vi "Initialize Scope and FGEN with Tclk.vi"(7 "Tclk Boolean Ref":refnum<vi>, 10 "FGEN Resources in":refnum<k15>[](array[refnum])=["FGEN1", "FGEN2"], 11 "Scope Resources in":refnum<k15>[](array[refnum])=["SCOPE1", "SCOPE2"]) -> (0 "error out":errorcluster, 1 "Tclk Refs Array":refnum<k20>[](array[refnum]), 2 "FGEN Resources out":refnum<k15>[](array[refnum]), 3 "Scope Resources out":refnum<k15>[](array[refnum]), 5 "scope channels":string[](array[string]))   [LabVIEW 2024]
uses:
  <instrlib>/niFgen/niFgen.llb/niFgen Output Mode.ctl
  <instrlib>/niFgen/niFgen.llb/niFgen Trigger Mode.ctl
  <instrlib>/niScope/Controls/niScope trigger source.ctl
  <instrlib>/niFgen/niFgen.llb/niFgen Create Waveform (WDT).vi
  <instrlib>/niScope/Configure/Trigger/niScope Configure Trigger Edge.vi
panel:
  out "Preparing T-Clk":bool
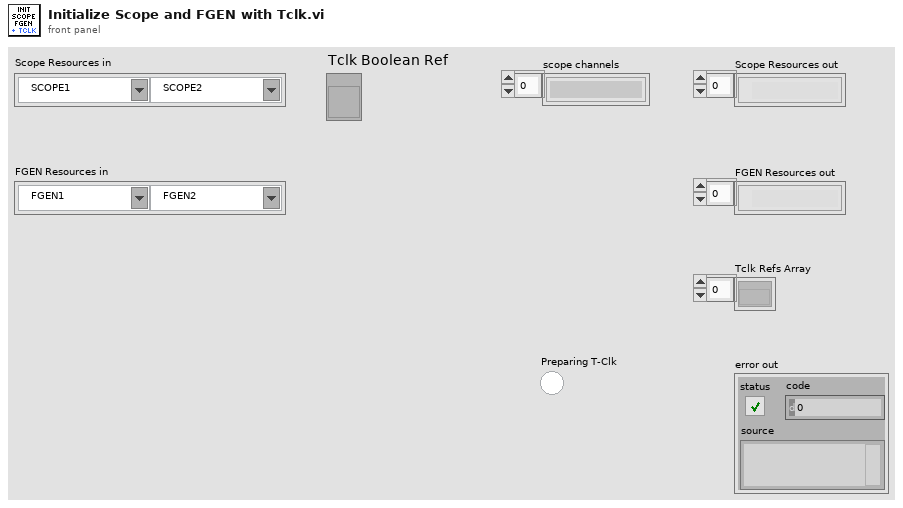
[diagram p1: front panel]
types:
  T1 = typedef "niScope trigger source.ctl" = string
  T2 = typedef "niFgen Trigger Mode.ctl" = i32
  T3 = typedef "niFgen Output Mode.ctl" = u32
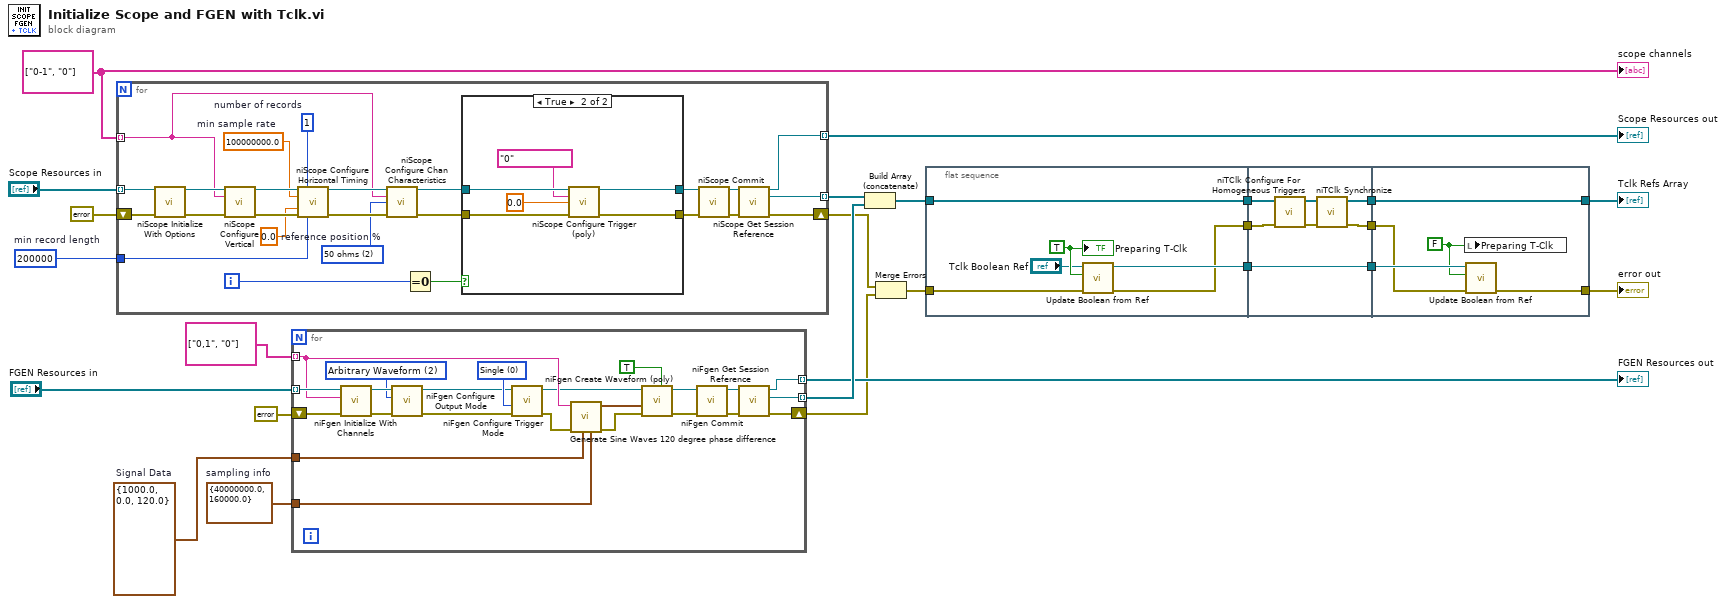
[diagram p0: block diagram]
diagram:
  w17 = 200000  # min record length
  w16 = cluster{"f":dbl, "startPhase":dbl, "dPhase":dbl} {"f"=1000.0, "startPhase"=0.0, "dPhase"=120.0}  # Signal Data
  w18 = cluster{"Fs":dbl, "#s":dbl} {"Fs"=40000000.0, "#s"=160000.0}  # sampling info
  w9 = string[] ["0-1", "0"] ("channels")
  n1 = for {
    tunnel: [w44] -> w15 mode=indexing
    tunnel: "Scope Resources in" -> [w35] mode=indexing
    tunnel: [w41] -> w6 mode=indexing
    tunnel: w9 -> [w27] mode=indexing
    shift-right: [w40] -> w1
    shift-left: errorcluster {"status"=FALSE, "code"=0, "source"=""} ("error out") -> [w39]
    tunnel: w17 -> [w26]
    i -> [w42]
    w28 = u32 2 items=["1 mega ohm"=0, "50 ohms"=2] ("input impedance")
    w36 = 0.0  # reference position %
    w37 = 1  # number of records
    w38 = 100000000.0  # min sample rate
    n2 = call <instrlib>:"niScope Initialize With Options.vi"("resource name"=w35, "error in"=w39) -> ("instrument handle"=w48:refnum<k15>, "error out"=w47:errorcluster)  [unwired: 12 in]
    n3 = call <instrlib>:"niScope Configure Vertical.vi"("instrument handle"=w48, "channels"=w27, "error in"=w47) -> ("instrument handle out"=w46:refnum<k15>, "error out"=w45:errorcluster)  [unwired: 11 in]
    n4 = call <instrlib>:"niScope Configure Horizontal Timing.vi"("instrument handle"=w46, "number of records"=w37, "min sample rate"=w38, "reference position"=w36, "error in"=w45, "min record length"=w26) -> ("instrument handle out"=w43:refnum<k15>, "error out"=w30:errorcluster)  [unwired: 8 in]
    n5 = call <instrlib>:"niScope Configure Chan Characteristics.vi"("instrument handle"=w43, "channels"=w27, "input impedance"=w28, "error in"=w30) -> ("instrument handle out"=w31:refnum<k15>, "error out"=w29:errorcluster)  [unwired: 10 in]
    n6 = Equal To 0?(x=w42) -> (x = 0?=w34:bool)
    n7 = case shown="True" w34 {
      tunnel: w31 -> [w52 w58]
      tunnel: w29 -> [w51 w57]
      tunnel: [w52 w56] -> w33
      tunnel: [w51 w55] -> w32
      frame False {
      }
      frame True {
        n8 = call-poly <instrlib>:"niScope Configure Trigger (poly).vi"("instrument handle"=w58, "trigger source"=T1 "0", "trigger level"=0.0, "error in"=w57) -> ("instrument handle out"=w56:refnum<k15>, "error out"=w55:errorcluster)  [unwired: 10 in]
      }
    }
    n9 = call <instrlib>:"niScope Commit.vi"("instrument handle"=w33, "error in"=w32) -> ("instrument handle out"=w50:refnum<k15>, "error out"=w49:errorcluster)  [unwired: 12 in]
    n10 = call <instrlib>:"niScope Get Session Reference.vi"("instrument handle"=w50, "error in"=w49) -> ("instrument handle out"=w41:refnum<k15>, "session reference"=w44:refnum<k20>, "error out"=w40:errorcluster)  [unwired: 11 in]
  }
  "Scope Resources out" <- w6
  n11 = for {
    tunnel: [w81] -> w14 mode=indexing
    tunnel: "FGEN Resources in" -> [w75] mode=indexing
    tunnel: [w80] -> w13 mode=indexing
    tunnel: string[] ["0,1", "0"] ("channels") -> [w70] mode=indexing
    shift-right: [w79] -> w7
    shift-left: errorcluster {"status"=FALSE, "code"=0, "source"=""} ("error out") -> [w76]
    tunnel: w18 -> [w65]
    tunnel: w16 -> [w64]
    w63 = T2 0 items=["Single", "Continuous", "Stepped", "Burst"] ("Trigger Mode (default: 1=continuous)")
    w72 = T3 2 items=["Standard Function", "Frequency List", "Arbitrary Waveform", "Arbitrary Sequence", "Script"] ("Output Mode (default: 0=Standard Function)")
    n12 = call <instrlib>:"niFgen Initialize With Channels.vi"("error in (no error)"=w76, "Channel Name"=w70, "Resource Name"=w75) -> ("error out"=w74:errorcluster, "Instrument Handle Out"=w73:refnum<k15>)  [unwired: 7 in]
    n13 = call <instrlib>:"niFgen Configure Output Mode.vi"("error in (no error)"=w74, "Output Mode (default: 0=Standard Function)"=w72, "Instrument Handle"=w73) -> ("error out"=w62:errorcluster, "Instrument Handle Out"=w61:refnum<k15>)  [unwired: 6 in]
    n14 = call <instrlib>:"niFgen Configure Trigger Mode.vi"("error in (no error)"=w62, "Trigger Mode (default: 1=continuous)"=w63, "Instrument Handle"=w61) -> ("error out"=w60:errorcluster, "Instrument Handle Out"=w59:refnum<k15>)  [unwired: 7 in]
    n15 = call "Generate Sine Waves 120 degree phase difference.vi"("sampling info"=w65, "Signal Data"=w64, "error in (no error)"=w60, "channels"=w70) -> ("error out"=w69:errorcluster, "signal out"=w68:waveform(dbl))  [unwired: 6 in]
    n16 = call-poly <instrlib>:"niFgen Create Waveform (poly).vi"("Use Waveform dT for Sample Rate"=TRUE, "error in (no error)"=w69, "Waveform"=w68, "Instrument Handle"=w59) -> ("error out"=w66:errorcluster, "Instrument Handle Out"=w67:refnum<k15>)  [unwired: 5 in, 1 out]
    n17 = call <instrlib>:"niFgen Commit.vi"("error in (no error)"=w66, "Instrument Handle"=w67) -> ("error out"=w78:errorcluster, "Instrument Handle Out"=w77:refnum<k15>)  [unwired: 8 in]
    n18 = call <instrlib>:"niFgen Get Session Reference.vi"("error in (no error)"=w78, "Instrument Handle"=w77) -> ("error out"=w79:errorcluster, "Session Reference"=w81:refnum<k20>, "Instrument Handle Out"=w80:refnum<k15>)  [unwired: 7 in]
  }
  "FGEN Resources out" <- w13
  n19 = Build Array (concatenate)(w15, w14) -> (w2:refnum<k20>[])
  n20 = Merge Errors(w1, w7) -> (w5:errorcluster)
  n21 = flat-sequence {
    tunnel: w5 -> [w83]
    tunnel: w2 -> [w87]
    tunnel: [w87] -> w25
    tunnel: [w82] -> w24
    tunnel: [w85] -> w23
    tunnel: [w91] -> w22
    tunnel: [w90] -> w21
    tunnel: w25 -> [w94]
    tunnel: w24 -> [w89]
    tunnel: [w88] -> w20
    tunnel: w23 -> [w88]
    tunnel: [w99] -> w3
    tunnel: w22 -> [w99]
    tunnel: w21 -> [w95]
    tunnel: w20 -> [w98]
    tunnel: [w96] -> w19
    frame #0 {
      w86 = TRUE
      n22 = call "Update Boolean from Ref.vi"("error in (no error)"=w83, "Boolean"=w86, "Boolean Ref in"="Tclk Boolean Ref") -> ("error out"=w82:errorcluster, "Boolean Ref out"=w85:refnum<vi>)  [unwired: 7 in]
      "Preparing T-Clk" <- w86
    }
    frame #1 {
      n23 = call <instrlib>:"niTClk Configure For Homogeneous Triggers.vi"("error in (no error)"=w89, "sessions"=w94) -> ("error out"=w92:errorcluster, "sessions out"=w93:refnum<k20>[])  [unwired: 8 in]
      n24 = call <instrlib>:"niTClk Synchronize.vi"("error in (no error)"=w92, "sessions"=w93) -> ("error out"=w90:errorcluster, "sessions out"=w91:refnum<k20>[])  [unwired: 8 in]
    }
    frame #2 {
      w97 = FALSE
      n25 = local write "Preparing T-Clk"(w97) -> ()
      n26 = call "Update Boolean from Ref.vi"("error in (no error)"=w95, "Boolean"=w97, "Boolean Ref in"=w98) -> ("error out"=w96:errorcluster)  [unwired: 7 in, 1 out]
    }
  }
  "error out" <- w19
  "scope channels" <- w9
  "Tclk Refs Array" <- w3
